vi "Upload Multiple Files.vi"(4 "attributes":refnum<class "File Attributes.lvclass">, 6 "timeout (ms)":i32=30000, 8 "error in":errorcluster, 10 "file specifications":T1[](array[typedef]), 11 "session in":refnum<class "Session.lvclass">) -> (0 "error out":errorcluster, 3 "session out":refnum<class "Session.lvclass">)   [LabVIEW 2020, in "NI_SFTP.lvlib"]
doc: "Creates multiple remote files."
uses:
  <vilib>/net/SFTP/NI_SFTP.lvlib
  <vilib>/net/SFTP/Session/Session.lvclass
  <vilib>/net/SFTP/API/Support/File Specification.ctl
  <vilib>/net/SFTP/File Attributes/File Attributes.lvclass
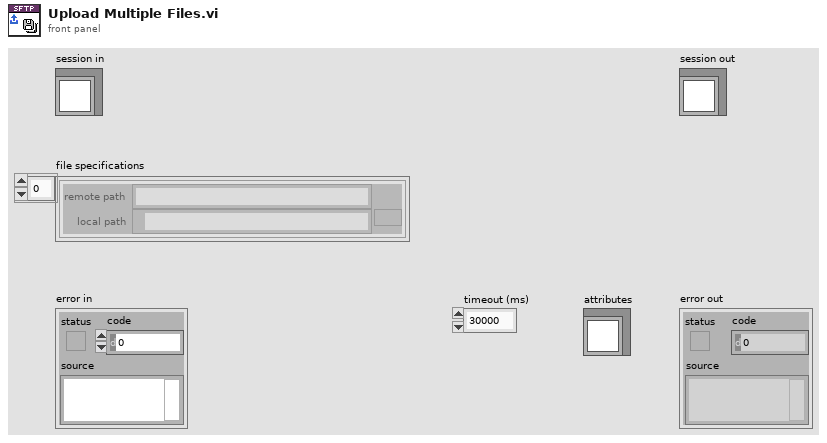
[diagram p1: front panel]
types:
  T1 = typedef "NI_SFTP.lvlib/File Specification.ctl" = cluster{"remote path":string, "local path":path}
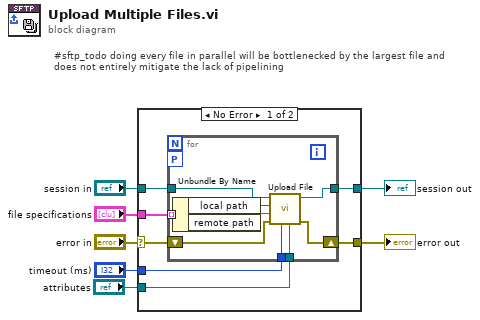
[diagram p0: block diagram]
diagram:
  # "#sftp_todo doing every file in parallel will be bottlenecked by the largest file and does not entirely mitigate the lack of pipelining"
  n1 = case shown="No Error" "error in" {
    selector: "error in" -> [w11 w25]
    tunnel: [w10 w25] -> w4
    tunnel: [w13 w24] -> w5
    tunnel: "session in" -> [w14 w24]
    tunnel: "timeout (ms)" -> [w12 _]
    tunnel: "file specifications" -> [w8 _]
    tunnel: "attributes" -> [w9 _]
    frame No Error {
      n2 = for {
        workers-P: _ -> [_]
        tunnel: w14 -> [w23]
        tunnel: [w21] -> w13
        tunnel: w12 -> [w19]
        shift-right: [w20] -> w10
        shift-left: w11 -> [w22]
        tunnel: w9 -> [w18]
        tunnel: w8 -> [w17] mode=indexing
        n3 = Unbundle By Name(w17) -> ("local path"=w16:path, "remote path"=w15:string)
        n4 = call <vilib>:"Upload File.vi"("attributes"=w18, "timeout (ms)"=w19, "error in"=w22, "remote path"=w15, "local path"=w16, "session in"=w23) -> ("error out"=w20:errorcluster, "session out"=w21:refnum<class "Session.lvclass">)  [unwired: 4 in]
      }
    }
    frame Error {
    }
  }
  "error out" <- w4
  "session out" <- w5
